vi "QC_MeasurementSetup.vi"() -> ()   [LabVIEW 2018]
uses:
  InstrControl/SupplyControl/SupplyControl.lvclass
  InstrControl/LCRControl/LCRControl.lvclass
  InstrControl/ArduinoControl/ArduinoControl.lvclass
  InstrControl/ProbeStationControl/ProbeStationControl.lvclass
  InstrControl/Switching/Switching.lvclass
  InstrControl/MultimeterControl/MultimeterControl.lvclass
panel:
  in  "Run Info":T1={"User"="", " Institute"="", " Test Time"="", " Test Date"="", "Instruments"="", "Sensor IDS"=[], "IV Test?"=TRUE, "CV Test? "=TRUE, "LCS Test? "=TRUE, "No. of Ch."=0, " Current Sensor"="", " Current Test"="", "Arduino DP Map"=["4", "5", "3", "2", "1", "0", "14", "15", "25", "23", "27", "29", "31", "33", "35", "37", "39", "43", "41", "45", "47", "49", "51", "53"], "Sensor BW"=[], "Sensor Types"=[], "Data directory"=""}
  in  "Hardware Settings":T2={"Supply"=refnum, "LCR"=refnum, "Arduino"=refnum, "Switching"=refnum, "SMU Name"="Keithley 2410", " LCR Name"="WayneKerr 6440B", " Volt Name "="Aglient 34401A", " Switching GPIB Address "="", "Temperature Readout"=enum."Read Arduino", "Voltmeter Visa"=""}
  in  "Ris Measurement Parameters":T3={"Bias Supply"=refnum, "SMU"=refnum, "Multimeter"=refnum, "Initial Voltage [V]"=20.0, "Final Voltage [V]"=-500.0, "Step Size [V]"=20.0, "Step Interval [s]"=10, "Number Of Steps"=25, "Ramp down steps [V]"=10.0, "Ramp down Interval [s]"=1, "Set Current Limit?"=TRUE, "Current Limit [µA]"=1000.0, "Temperature Readout"=enum."Read Arduino", "Arduino"=refnum, "Supply Name"="Keithley 487", "SMU Name"="Keithley 6517", "Voltmeter Name"="Keithley 2000", "R_is Limit [MOhm]"=-500.0, "Switching"=refnum, "Matrix used?"=FALSE, "Matrix X Channels"={"Bias Supply / SMU LO"=5, "Bias Supply / SMU HI"=6, "CV Box LO"=3, "CV Box HI"=4, "CV Box LO IN"=7, "CV Box HI IN"=8, "Volt meter LO"=1, "Volt meter HI"=2, "Mux1 C1"=9, "Mux1 C2"=10, "Mux2 C1"=11, "Mux2 C2"=12}} {"Current Limit [µA]" format="%.3f"; "Step Size [V]" format="%.1f"; "Final Voltage [V]" format="%.1f"; "Initial Voltage [V]" format="%.1f"}
  in  "Current Stability Measurement Parameters":T4={"Supply"=refnum, "Voltage [V]"=-700.0, "Measurement Interval [s]"=10, "Test Duration"=86400, "Ramp up steps [V]"=10.0, "Ramp up Interval [s]"=1, "Ramp down steps [V]"=50.0, "Ramp down Interval [s]"=1, "Set Current Limit?"=TRUE, "Current Limit [µA]"=1000.0, "Temperature Readout"=enum."Read Arduino", "Arduino"=refnum, "Supply Name"="", "Maximum current fluctuation [%]"=2.0, "Switching.lvclass"=refnum, "Matrix used?"=FALSE, "Matrix X Channels"={"Bias Supply / SMU LO"=5, "Bias Supply / SMU HI"=6, "CV Box LO"=3, "CV Box HI"=4, "CV Box LO IN"=7, "CV Box HI IN"=8, "Volt meter LO"=1, "Volt meter HI"=2, "Mux1 C1"=9, "Mux1 C2"=10, "Mux2 C1"=11, "Mux2 C2"=12}, "LCS Test?"=TRUE, "Number of Steps"=10, "Norm. to Temp."=0.0} {"Current Limit [µA]" format="%.3f"; "Test Duration" format="%<%H:%M:%S>t"; "Voltage [V]" format="%.1f"}
  in  "Cis Measurement Parameters":T5={"Supply"=refnum, "LCR"=refnum, "Initial Voltage [V]"=0.0, "Final Voltage [V]"=-700.0, "Step Size [V]"=10.0, "Step Interval [s]"=5, "Number Of Steps"=71, "AC frequency [Hz]"=100000, "RC Configuration"=1, "AC amplitude [V]"=0.1, "Ramp down steps [V]"=10.0, "Ramp down Interval [s]"=1, "Set Current Limit?"=TRUE, "Current Limit [µA]"=1000.0, "Temperature Readout"=enum."Read Arduino", "Arduino"=refnum, "Supply Name"="", "LCR Name"="", "C_is Limit [pF/cm]"=1.0, "Switching"=refnum, "Matrix used?"=FALSE, "Matrix X Channels"={"Bias Supply / SMU LO"=5, "Bias Supply / SMU HI"=6, "CV Box LO"=3, "CV Box HI"=4, "CV Box LO IN"=7, "CV Box HI IN"=8, "Volt meter LO"=1, "Volt meter HI"=2, "Mux1 C1"=9, "Mux1 C2"=10, "Mux2 C1"=11, "Mux2 C2"=12}} {"Current Limit [µA]" format="%.3f"; "RC Configuration" items=["serial", "parallel"]; "Step Size [V]" format="%.1f"; "Final Voltage [V]" format="%.1f"; "Initial Voltage [V]" format="%.1f"}
  in  "CV Measurement Parameters":T6={"Supply"=refnum, "LCR"=refnum, "Initial Voltage [V]"=0.0, "Final Voltage [V]"=-700.0, "Step Size [V]"=10.0, "Step Interval [s]"=5, "Number Of Steps"=71, "AC frequency [Hz]"=500, "RC Configuration"=0, "AC amplitude [V]"=0.1, "Ramp down steps [V]"=10.0, "Ramp down Interval [s]"=1, "Set Current Limit?"=TRUE, "Current Limit [µA]"=1000.0, "Temperature Readout"=enum."Read Arduino", "Arduino"=refnum, "Supply Name"="", "LCR Name"="", "V_depletion Limit [V]"=-300.0, "Switching"=refnum, "Matrix used?"=FALSE, "Matrix X Channels"={"Bias Supply / SMU LO"=5, "Bias Supply / SMU HI"=6, "CV Box LO"=3, "CV Box HI"=4, "CV Box LO IN"=7, "CV Box HI IN"=8, "Volt meter LO"=1, "Volt meter HI"=2, "Mux1 C1"=9, "Mux1 C2"=10, "Mux2 C1"=11, "Mux2 C2"=12}, "CV Test?"=TRUE} {"Current Limit [µA]" format="%.3f"; "RC Configuration" items=["serial", "parallel"]; "Step Size [V]" format="%.1f"; "Final Voltage [V]" format="%.1f"; "Initial Voltage [V]" format="%.1f"}
  in  "IV Measurement Parameters":T7={"Supply"=refnum, "Initial Voltage [V]"=0.0, "Final Voltage [V]"=-700.0, "Step Size [V]"=10.0, "Step Interval [s]"=10, "Number Of Steps"=71, "Ramp down steps [V]"=50.0, "Ramp down Interval [s]"=1, "hold steps"=6, "Set Current Limit?"=TRUE, "Current Limit [µA]"=1000.0, "Temperature Readout"=enum."Read Arduino", "Arduino"=refnum, "Supply Name"="", "V_breakdown Limit [V]"=0.0, "Switching"=refnum, "Matrix used?"=FALSE, "Matrix X Channels"={"Bias Supply / SMU LO"=5, "Bias Supply / SMU HI"=6, "CV Box LO"=3, "CV Box HI"=4, "CV Box LO IN"=7, "CV Box HI IN"=8, "Volt meter LO"=1, "Volt meter HI"=2, "Mux1 C1"=9, "Mux1 C2"=10, "Mux2 C1"=11, "Mux2 C2"=12}, "IV Test?"=TRUE} {"Current Limit [µA]" format="%.3f"; "Step Size [V]" format="%.1f"; "Final Voltage [V]" format="%.1f"; "Initial Voltage [V]" format="%.1f"}
  in  "Striptest Measurement Parameters":T8={"Bias Supply"=refnum, "SMU"=refnum, "LCR"=refnum, "Probe Card Channels"=32, "Bias Voltage [V]"=-150.0, "First strip"=1, "Last strip"=1280, "Base Voltage [V]"=10.0, "Base Ramp Step [V]"=10.0, "Base Ramp Interval [ms]"=1000, "High Voltage [V]"=100.0, "High Ramp Step [V]"=100.0, "High Ramp Interval [ms]"=1000, "AC frequency [Hz]"=100000, "AC amplitude [V]"=0.1, "RC Configuration"=0, "Single Needle"=FALSE, "Temperature Readout"=enum."Read Arduino", "Arduino"=refnum, "Fraction of good strips [%]"=98.0, "ProbeStation"=refnum, "Switching"=refnum, "Matrix used?"=FALSE, "Matrix X Channels"={"Bias Supply / SMU LO"=5, "Bias Supply / SMU HI"=6, "CV Box LO"=3, "CV Box HI"=4, "CV Box LO IN"=7, "CV Box HI IN"=8, "Volt meter LO"=1, "Volt meter HI"=2, "Mux1 C1"=9, "Mux1 C2"=10, "Mux2 C1"=11, "Mux2 C2"=12}, "Pinholes Y/N"=TRUE, "Capacitance Y/N"=TRUE, "Resistance Y/N"=TRUE, "Bias Supply Name"="", "SMU Name"="", "LCR Name"=""} {"RC Configuration" items=["serial", "parallel"]; "High Ramp Step [V]" format="%.1f"; "High Voltage [V]" format="%.1f"; "Base Ramp Step [V]" format="%.1f"; "Base Voltage [V]" format="%.1f"; "Bias Voltage [V]" format="%.1f"}
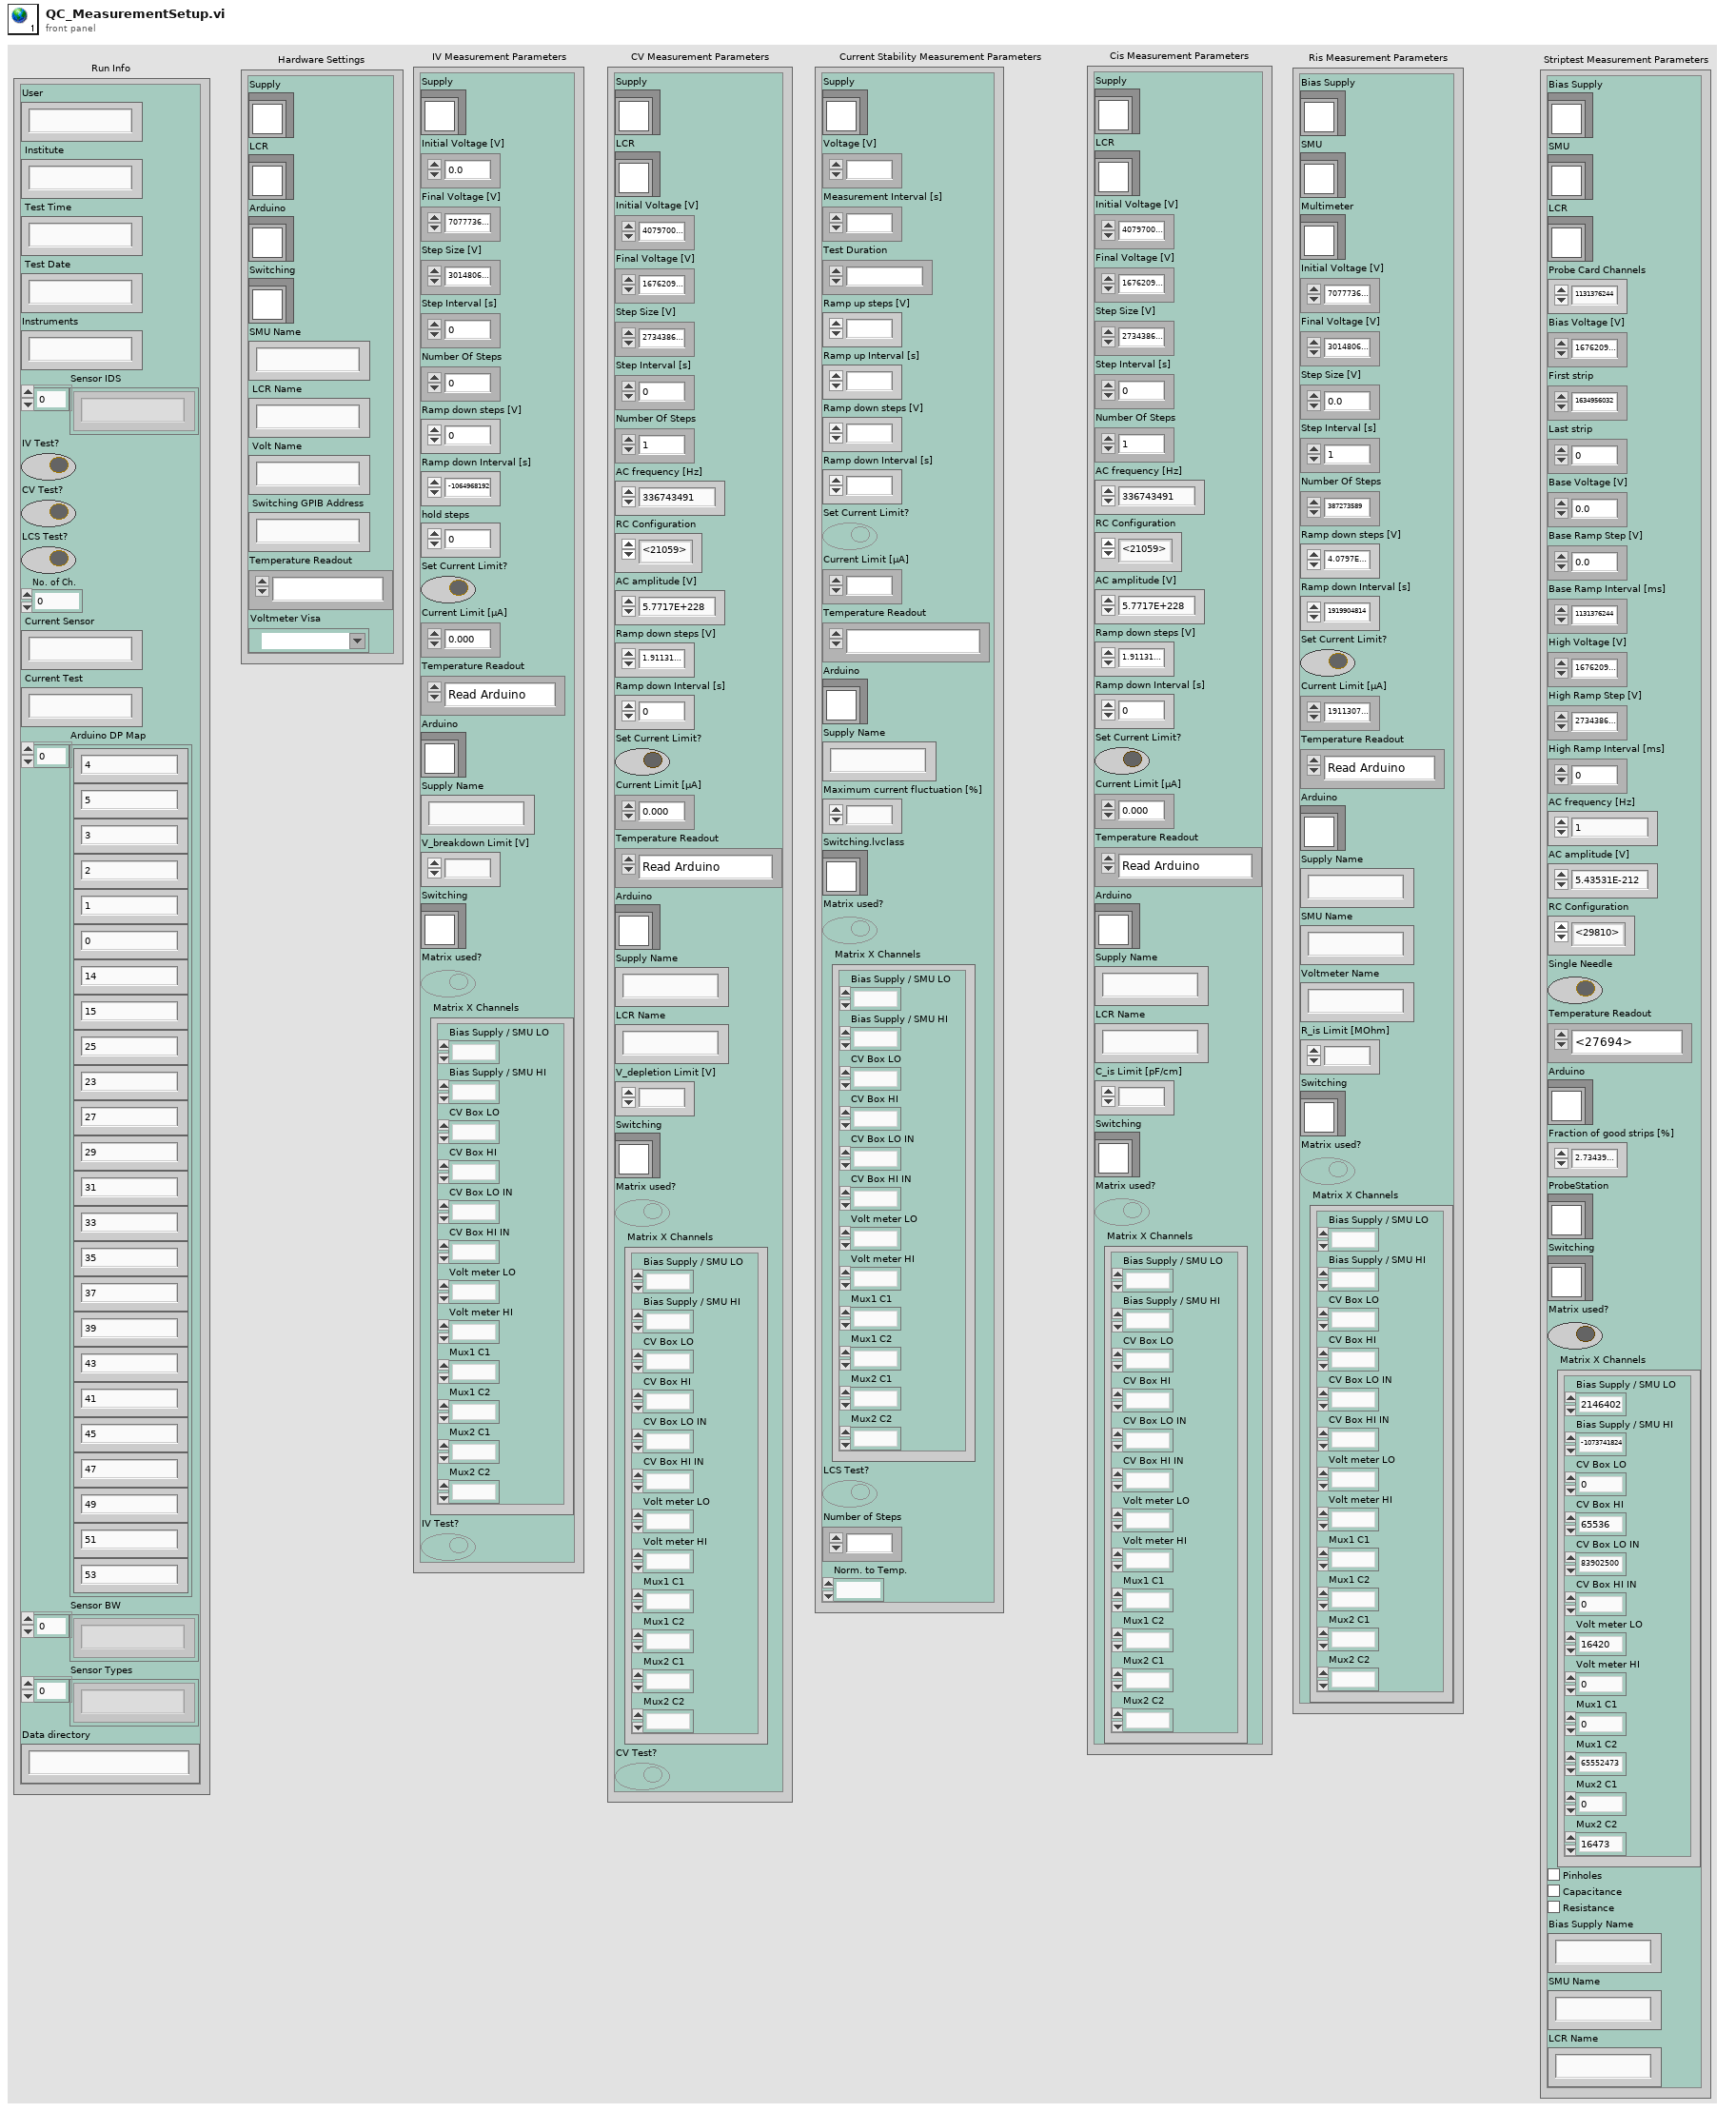
[diagram p1: front panel]
types:
  T1 = cluster{"User":string, " Institute":string, " Test Time":string, " Test Date":string, "Instruments":string, "Sensor IDS":string[], "IV Test?":bool, "CV Test? ":bool, "LCS Test? ":bool, "No. of Ch.":u16, " Current Sensor":string, " Current Test":string, "Arduino DP Map":string[], "Sensor BW":string[], "Sensor Types":string[], "Data directory":string}
  T2 = cluster{"Supply":refnum<class "SupplyControl.lvclass">, "LCR":refnum<class "LCRControl.lvclass">, "Arduino":refnum<class "ArduinoControl.lvclass">, "Switching":refnum<class "Switching.lvclass">, "SMU Name":string, " LCR Name":string, " Volt Name ":string, " Switching GPIB Address ":string, "Temperature Readout":enum16{"Read Arduino", "Enter manually"}, "Voltmeter Visa":refnum<visa-resource-name>}
  T3 = cluster{"Bias Supply":refnum<class "SupplyControl.lvclass">, "SMU":refnum<class "SupplyControl.lvclass">, "Multimeter":refnum<class "MultimeterControl.lvclass">, "Initial Voltage [V]":dbl, "Final Voltage [V]":dbl, "Step Size [V]":dbl, "Step Interval [s]":i32, "Number Of Steps":u32, "Ramp down steps [V]":dbl, "Ramp down Interval [s]":i32, "Set Current Limit?":bool, "Current Limit [µA]":dbl, "Temperature Readout":enum16{"Read Arduino", "Enter manually"}, "Arduino":refnum<class "ArduinoControl.lvclass">, "Supply Name":string, "SMU Name":string, "Voltmeter Name":string, "R_is Limit [MOhm]":dbl, "Switching":refnum<class "Switching.lvclass">, "Matrix used?":bool, "Matrix X Channels":cluster{"Bias Supply / SMU LO":i32, "Bias Supply / SMU HI":i32, "CV Box LO":i32, "CV Box HI":i32, "CV Box LO IN":i32, "CV Box HI IN":i32, "Volt meter LO":i32, "Volt meter HI":i32, "Mux1 C1":i32, "Mux1 C2":i32, "Mux2 C1":i32, "Mux2 C2":i32}}
  T4 = cluster{"Supply":refnum<class "SupplyControl.lvclass">, "Voltage [V]":dbl, "Measurement Interval [s]":i32, "Test Duration":u32, "Ramp up steps [V]":dbl, "Ramp up Interval [s]":u32, "Ramp down steps [V]":dbl, "Ramp down Interval [s]":i32, "Set Current Limit?":bool, "Current Limit [µA]":dbl, "Temperature Readout":enum16{"Read Arduino", "Enter manually"}, "Arduino":refnum<class "ArduinoControl.lvclass">, "Supply Name":string, "Maximum current fluctuation [%]":dbl, "Switching.lvclass":refnum<class "Switching.lvclass">, "Matrix used?":bool, "Matrix X Channels":cluster{"Bias Supply / SMU LO":i32, "Bias Supply / SMU HI":i32, "CV Box LO":i32, "CV Box HI":i32, "CV Box LO IN":i32, "CV Box HI IN":i32, "Volt meter LO":i32, "Volt meter HI":i32, "Mux1 C1":i32, "Mux1 C2":i32, "Mux2 C1":i32, "Mux2 C2":i32}, "LCS Test?":bool, "Number of Steps":i32, "Norm. to Temp.":dbl}
  T5 = cluster{"Supply":refnum<class "SupplyControl.lvclass">, "LCR":refnum<class "LCRControl.lvclass">, "Initial Voltage [V]":dbl, "Final Voltage [V]":dbl, "Step Size [V]":dbl, "Step Interval [s]":i32, "Number Of Steps":u32, "AC frequency [Hz]":i32, "RC Configuration":u16, "AC amplitude [V]":dbl, "Ramp down steps [V]":dbl, "Ramp down Interval [s]":i32, "Set Current Limit?":bool, "Current Limit [µA]":dbl, "Temperature Readout":enum16{"Read Arduino", "Enter manually"}, "Arduino":refnum<class "ArduinoControl.lvclass">, "Supply Name":string, "LCR Name":string, "C_is Limit [pF/cm]":dbl, "Switching":refnum<class "Switching.lvclass">, "Matrix used?":bool, "Matrix X Channels":cluster{"Bias Supply / SMU LO":i32, "Bias Supply / SMU HI":i32, "CV Box LO":i32, "CV Box HI":i32, "CV Box LO IN":i32, "CV Box HI IN":i32, "Volt meter LO":i32, "Volt meter HI":i32, "Mux1 C1":i32, "Mux1 C2":i32, "Mux2 C1":i32, "Mux2 C2":i32}}
  T6 = cluster{"Supply":refnum<class "SupplyControl.lvclass">, "LCR":refnum<class "LCRControl.lvclass">, "Initial Voltage [V]":dbl, "Final Voltage [V]":dbl, "Step Size [V]":dbl, "Step Interval [s]":i32, "Number Of Steps":u32, "AC frequency [Hz]":i32, "RC Configuration":u16, "AC amplitude [V]":dbl, "Ramp down steps [V]":dbl, "Ramp down Interval [s]":i32, "Set Current Limit?":bool, "Current Limit [µA]":dbl, "Temperature Readout":enum16{"Read Arduino", "Enter manually"}, "Arduino":refnum<class "ArduinoControl.lvclass">, "Supply Name":string, "LCR Name":string, "V_depletion Limit [V]":dbl, "Switching":refnum<class "Switching.lvclass">, "Matrix used?":bool, "Matrix X Channels":cluster{"Bias Supply / SMU LO":i32, "Bias Supply / SMU HI":i32, "CV Box LO":i32, "CV Box HI":i32, "CV Box LO IN":i32, "CV Box HI IN":i32, "Volt meter LO":i32, "Volt meter HI":i32, "Mux1 C1":i32, "Mux1 C2":i32, "Mux2 C1":i32, "Mux2 C2":i32}, "CV Test?":bool}
  T7 = cluster{"Supply":refnum<class "SupplyControl.lvclass">, "Initial Voltage [V]":dbl, "Final Voltage [V]":dbl, "Step Size [V]":dbl, "Step Interval [s]":i32, "Number Of Steps":u32, "Ramp down steps [V]":dbl, "Ramp down Interval [s]":i32, "hold steps":i32, "Set Current Limit?":bool, "Current Limit [µA]":dbl, "Temperature Readout":enum16{"Read Arduino", "Enter manually"}, "Arduino":refnum<class "ArduinoControl.lvclass">, "Supply Name":string, "V_breakdown Limit [V]":dbl, "Switching":refnum<class "Switching.lvclass">, "Matrix used?":bool, "Matrix X Channels":cluster{"Bias Supply / SMU LO":i32, "Bias Supply / SMU HI":i32, "CV Box LO":i32, "CV Box HI":i32, "CV Box LO IN":i32, "CV Box HI IN":i32, "Volt meter LO":i32, "Volt meter HI":i32, "Mux1 C1":i32, "Mux1 C2":i32, "Mux2 C1":i32, "Mux2 C2":i32}, "IV Test?":bool}
  T8 = cluster{"Bias Supply":refnum<class "SupplyControl.lvclass">, "SMU":refnum<class "SupplyControl.lvclass">, "LCR":refnum<class "LCRControl.lvclass">, "Probe Card Channels":i32, "Bias Voltage [V]":dbl, "First strip":i32, "Last strip":i32, "Base Voltage [V]":dbl, "Base Ramp Step [V]":dbl, "Base Ramp Interval [ms]":u32, "High Voltage [V]":dbl, "High Ramp Step [V]":dbl, "High Ramp Interval [ms]":u32, "AC frequency [Hz]":i32, "AC amplitude [V]":dbl, "RC Configuration":u16, "Single Needle":bool, "Temperature Readout":enum16{"Read Arduino", "Enter manually"}, "Arduino":refnum<class "ArduinoControl.lvclass">, "Fraction of good strips [%]":dbl, "ProbeStation":refnum<class "ProbeStationControl.lvclass">, "Switching":refnum<class "Switching.lvclass">, "Matrix used?":bool, "Matrix X Channels":cluster{"Bias Supply / SMU LO":i32, "Bias Supply / SMU HI":i32, "CV Box LO":i32, "CV Box HI":i32, "CV Box LO IN":i32, "CV Box HI IN":i32, "Volt meter LO":i32, "Volt meter HI":i32, "Mux1 C1":i32, "Mux1 C2":i32, "Mux2 C1":i32, "Mux2 C2":i32}, "Pinholes Y/N":bool, "Capacitance Y/N":bool, "Resistance Y/N":bool, "Bias Supply Name":string, "SMU Name":string, "LCR Name":string}
diagram:
